vi "DS345.ProcPeriodic.vi"(0 "i ref in":refnum<vi>, 3 "timeout [ms] (10000)":i32=10000, 5 "error in (no error)":errorcluster) -> (14 "i ref out":refnum<vi>, 17 "timed out":bool, 19 "error out":errorcluster)   [LabVIEW 2014, in "DS345.lvlib"]
doc: "This method serves to periodically do things like reading values from the HW. Methods that should be executed periodically should be called from THIS method. Add code here."
uses:
  DS345.lvlib
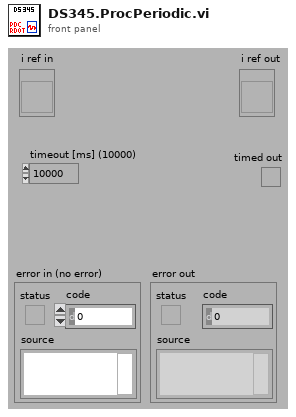
[diagram p1: front panel]
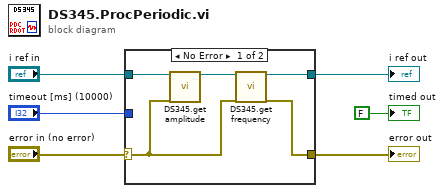
[diagram p0: block diagram]
diagram:
  n1 = case shown="No Error" "error in (no error)" {
    selector: "error in (no error)" -> [w8 w12]
    tunnel: "i ref in" -> [w11 w13]
    tunnel: [w7 w12] -> w5
    tunnel: [w9 w13] -> w4
    tunnel: "timeout [ms] (10000)" -> [_ _]
    frame No Error {
      n2 = call "DS345.get amplitude.vi"("i ref in"=w11, "error in (no error)"=w8) -> ("i ref out"=w10:refnum<vi>)  [unwired: 15 in, 2 out]
      n3 = call "DS345.get frequency.vi"("i ref in"=w10, "error in (no error)"=w8) -> ("i ref out"=w9:refnum<vi>, "error out"=w7:errorcluster)  [unwired: 15 in, 1 out]
    }
    frame Error {
    }
  }
  "error out" <- w5
  "i ref out" <- w4
  "timed out" <- FALSE ("timed out")
